vi "Mirror Image(24bit Horizontal).vi"(8 "错误输入":errorcluster, 11 "image In":T1 caption="Image in") -> (0 "错误输出":errorcluster, 3 "image out":T1 caption="Image out")   [LabVIEW 2012, in "Picture Box Tools.lvlib"]
uses:
  <vilib>/picture/picture.llb/imagedata.ctl
  Picture Box Tools.lvlib
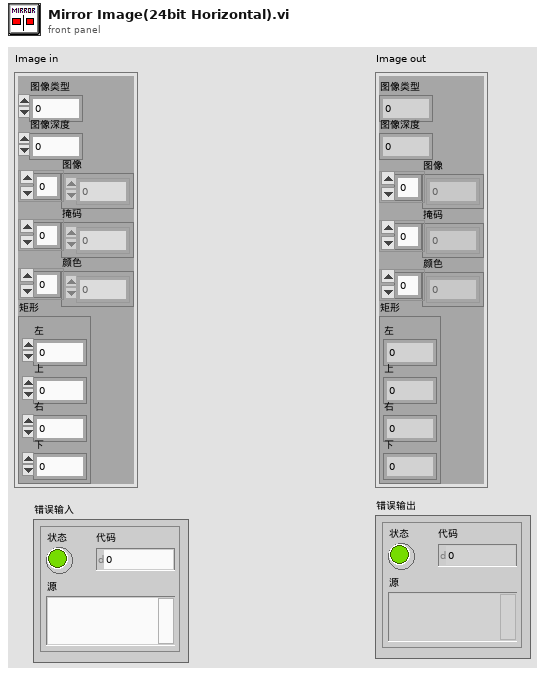
[diagram p1: front panel]
types:
  T1 = typedef "imagedata.ctl" = cluster{"image type":i32, "image depth":i32, "image":u8[], "mask":u8[], "colors":u32[], "Rectangle":cluster{"left":i16, "top":i16, "right":i16, "bottom":i16}}
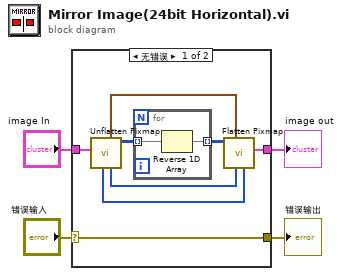
[diagram p0: block diagram]
diagram:
  n1 = case shown="无错误" "错误输入" {
    selector: "错误输入" -> [w7 w15]
    tunnel: [w7 w15] -> w3
    tunnel: "image In" -> [w6 _]
    tunnel: [w5 _] -> w1
    frame No Error {
      n2 = call <vilib>:"Unflatten Pixmap.vi"("image data"=w6) -> ("24-bit pixmap"=w12:u32[][], "colors"=w10:u32[], "top left"=w8:cluster{"x":i16, "y":i16}, "mask"=w9:u8[])  [unwired: 4 in, 3 out]
      n3 = for {
        tunnel: w12 -> [w14] mode=indexing
        tunnel: [w13] -> w11 mode=indexing
        n4 = Reverse 1D Array(array=w14) -> (reversed array=w13:u32[])
      }
      n5 = call <vilib>:"Flatten Pixmap.vi"("mask"=w9, "colors"=w10, "top left"=w8, "24-bit pixmap"=w11) -> ("image data"=w5:T1)  [unwired: 7 in]
    }
    frame Error {
    }
  }
  "错误输出" <- w3
  "image out" <- w1
